vi "FilterRequests.vi"() -> ()   [LabVIEW 2015]
uses:
  TypeDef/RequestsTableColumnNamesRing.ctl
  TypeDef/RequestTableCluster.ctl
panel:
  in  "From":timestamp
  in  "To":timestamp
  in  "Filter Text":string
  out "Requests":T1[](array[typedef])
  in  "Filter 1":T2
  out "error out":errorcluster
  in  "error in":errorcluster
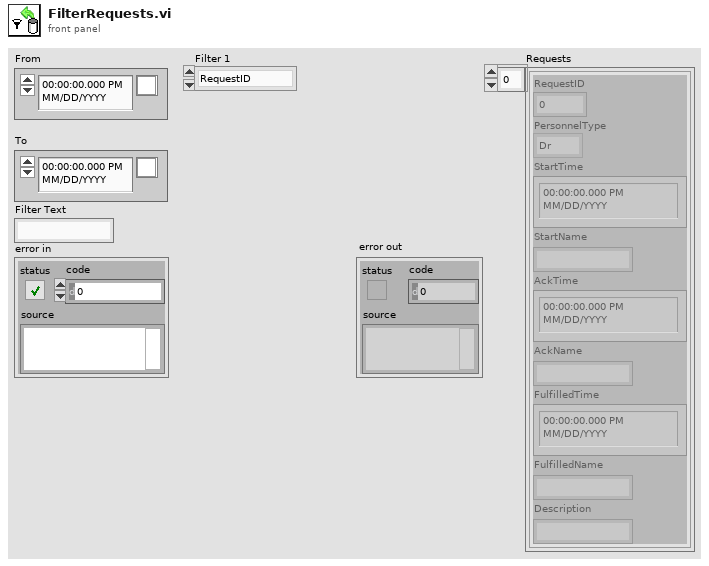
[diagram p1: front panel]
types:
  T1 = typedef "RequestTableCluster.ctl" = cluster{"RequestID":u32, "PersonnelType":enum16{"Dr", "Nurse"}, "StartTime":timestamp, "StartName":string, "AckTime":timestamp, "AckName":string, "FulfilledTime":timestamp, "FulfilledName":string, "Description":string}
  T2 = typedef "RequestsTableColumnNamesRing.ctl" = enum16{"RequestID", "PersonnelType", "StartTime", "StartName", "AckTime", "AckName", "FulfilledTime", "FulfilledName", "Description"}
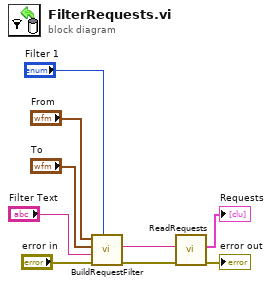
[diagram p0: block diagram]
diagram:
  n1 = call "BuildRequestFilter.vi"("Filter"="Filter 1", "error in"="error in", "Filter Text"="Filter Text", "To"="To", "From"="From") -> ("error out"=w7:errorcluster, "condition"=w5:string)  [unwired: 4 in, 1 out]
  n2 = call "ReadRequests.vi"("error in"=w7, "condition"=w5) -> ("error out"=→"error out":errorcluster, "Requests"=→"Requests":T1[])  [unwired: 8 in]
